vi "niLvFpga_AcquireWriteRegionFifo_cRIO-9035.vi"(0 "session in":u32, 1 "scalarType":u32, 2 "bitWidth":u32, 5 "Channel":u32, 7 "Empty Ref In":refnum<data-value>, 9 "Number Of Elements":u32, 11 "error in":errorcluster, 12 "Timeout(ms)":i32=-1) -> (4 "session out":u32, 6 "elementsInRegion":u32, 8 "writeRegionReference":refnum<data-value>, 10 "elementsRemaining":u32, 15 "error out":errorcluster)   [LabVIEW 2017]
doc: "Performance related peculiarities:\n\n1. Disable the Call Library Function's \"Generate Wrappers\" feature. This feature is displayed when you add the following labview.ini token, and right click on the Call Library Function node:\nextFuncGenNoWrapperEnabled=True\n\n2. For the Call Library function, enable \"Constant\" for parameters >> session.\n\n3. Remove the error case structure around the Call Library Functions. Chaining the errors between multiple Call Library Functions will suffice."
uses:
  <vilib>/rvi/errors/niLvFpgaWhatHappensToTopLevelVI.ctl
  <vilib>/rvi/interface/common/niFpgaNodeNameForErrorReporting.ctl
  NiFpgaLv.dll
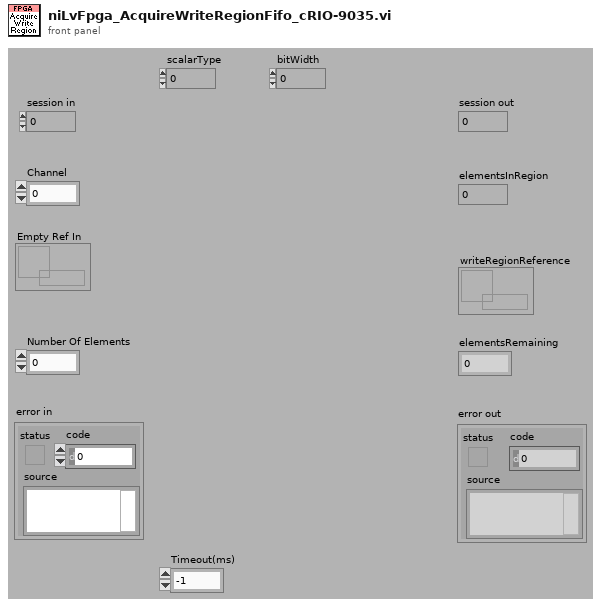
[diagram p1: front panel]
types:
  T1 = typedef "niFpgaNodeNameForErrorReporting.ctl" = enum16{"Open FPGA VI Reference", "Read/Write Control", "Invoke Method: Abort", "Invoke Method: Acknowledge IRQ", "Invoke Method: Download", "Invoke Method: FIFO.Configure", "Invoke Method: FIFO.Read", "Invoke Method: FIFO.Start", "Invoke Method: FIFO.Stop", "Invoke Method: FIFO.Write", "Invoke Method: Reset", "Invoke Method: Run", "Invoke Method: Wait on IRQ", "Close FPGA VI Reference", "Invoke Method: FIFO.Acquire Read Region", "Invoke Method: FIFO.Acquire Write Region"}
  T2 = typedef "niLvFpgaWhatHappensToTopLevelVI.ctl" = enum16{"top level VI scripted behind XNode", "top level VI inlined behind XNode"}
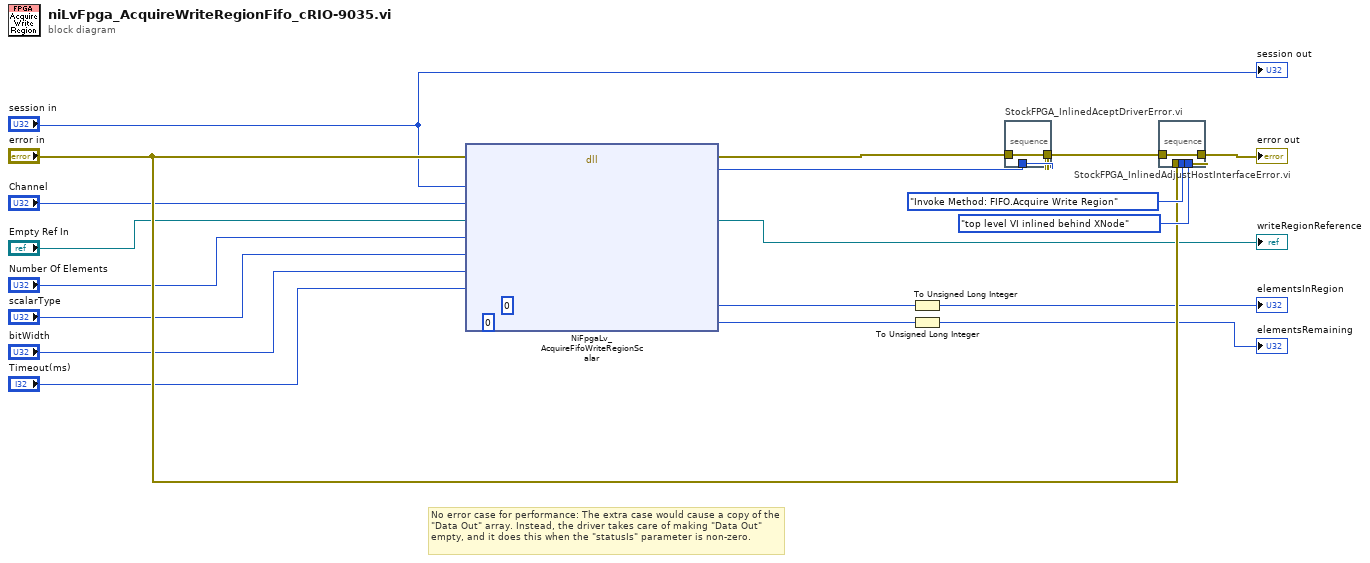
[diagram p0: block diagram]
diagram:
  # "No error case for performance: The extra case would cause a copy of the \"Data Out\" array. Instead, the driver takes care of making \"Data Out\" empty, and it does this when the \"statusIs\" parameter is non-zero."
  n1 = dll-call lib="NiFpgaLv.*" fn="NiFpgaLv_AcquireFifoWriteRegionScalar" label="niLvFpgaAcquireWriteRegionFifo"(error in="error in", "session"="session in", "channel"="Channel", "writeRegionReference"="Empty Ref In", "numberOfElements"="Number Of Elements", "scalarType"="scalarType", "bitWidth"="bitWidth", "timeout"="Timeout(ms)", "elementsInRegion"=u64 0, "elementsRemaining"=u64 0) -> (error out=w19:errorcluster, "status"=w17:i32, "writeRegionReference"=→"writeRegionReference":refnum<data-value>, "elementsInRegion"=w6:u64, "elementsRemaining"=w5:u64)  [unwired: 8 in, 1 out]
  n2 = To Unsigned Long Integer(number=w6) -> (unsigned 32bit integer=→"elementsInRegion":u32)
  n3 = To Unsigned Long Integer(number=w5) -> (unsigned 32bit integer=→"elementsRemaining":u32)
  n4 = stacked-sequence "StockFPGA_InlinedAceptDriverError.vi" {
    tunnel: w19 -> [w22]
    tunnel: w17 -> [w24]
    tunnel: [w23] -> w18
    frame #0 {
      n5 = case shown="Default" w24 {
        selector: w24 -> [_ w26]
        tunnel: [w25 w28] -> w23
        tunnel: w22 -> [w25 w29]
        frame 0 {
        }
        frame Default {
          n6 = Greater Than 0?(x=w26) -> (x > 0?=w27:bool)
          n7 = call <vilib>:"Error Cluster From Error Code.vi"("is warning? (False)"=w27, "error in (no error)"=w29, "error code (0)"=w26) -> ("error out"=w28:errorcluster)  [unwired: 6 in]
        }
      }
    }
  }
  n8 = stacked-sequence "StockFPGA_InlinedAdjustHostInterfaceError.vi" {
    tunnel: w18 -> [w35]
    tunnel: "error in" -> [w32]
    tunnel: niFpgaNodeNameForErrorReporting."Invoke Method: FIFO.Acquire Write Region" ("node name for error reporting") -> [w30]
    tunnel: niLvFpgaWhatHappensToTopLevelVI."top level VI inlined behind XNode" ("what happens to top level VI") -> [w31]
    tunnel: [w33] -> w8
    frame #0 {
      n9 = Unbundle By Name(w35) -> ("code"=w34:i32)
      n10 = case shown="Default" w34 {
        tunnel: [w36 w41] -> w33
        tunnel: w32 -> [w36 w40]
        tunnel: w31 -> [_ w39]
        tunnel: w30 -> [_ w38]
        tunnel: w35 -> [_ w37]
        frame 0 {
        }
        frame Default {
          n11 = call <vilib>:"niLvFpgaAdjustHostInterfaceError.vi"("error in"=w37, "prior error in"=w40, "node name for error reporting"=w38, "what happens to top level VI"=w39) -> ("error out"=w41:errorcluster)  [unwired: 11 in]
        }
      }
    }
  }
  "error out" <- w8
  "session out" <- "session in"
